vi "Instrument_IO Shift Variables.vi"(8 "error in":errorcluster, 11 "Main Config File Refnum":T1) -> (0 "error out":errorcluster, 3 "VARS Instrument_IO":T2={"error"={"status"=FALSE, "code"=0, "source"=""}, "AI_Tasks_State"=enum."Idle", "AO_Tasks_State"=enum."Idle", "RUN_PMT_AI"=FALSE, "RUN_PMT_AO"=FALSE, "RUN_PMT_DI"=FALSE, "WDT Time Stamp 1"=timestamp(0 s since 1904-01-01), "WDT Time Stamp 2"=timestamp(0 s since 1904-01-01), "RT_TO"=0, "WDT_TO"=0.0, "AO Tasks"=[], "DI Tasks"=[], "Tag Set Directory"=path "c:/ni-rt/startup/tagset", "LogPath"=path "", "DI_Tasks_State"=enum."Idle", "DO Tasks"=[], "RUN_PMT_DO"=FALSE, "DO_Tasks_State"=enum."Idle", "LogErrors?"=FALSE, "System Type"="", "AI Sample Rate"=0.0, "Timed Loop Rate"=0.0, "AI Averaging On"=FALSE, "Agilent Visa Resource"="Agilent", "FEM Visa Resource"="Agilent", "AI Tasks"=""} {"WDT_TO" format="%_4g"})   [LabVIEW 2018]
uses:
  Instrument_IO Shift Variables.ctl
  Common/Module Manager/MM_Module_Action.ctl
  <vilib>/Utility/config.llb/Config Data RefNum.ctl
  Common/COMM_Queues/Command Queue Cluster.ctl
  <vilib>/Utility/config.llb/Read Key (Double).vi
  <vilib>/Utility/config.llb/Read Key (String).vi
  <vilib>/Utility/config.llb/NI_LVConfig.lvlib
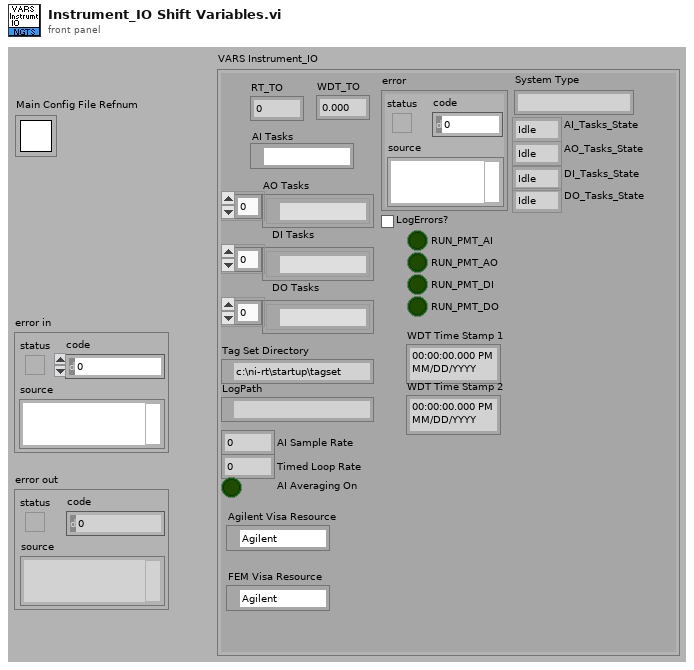
[diagram p1: front panel]
types:
  T1 = typedef "NI_LVConfig.lvlib/Config Data RefNum.ctl" = refnum<k1>
  T2 = typedef "Instrument_IO Shift Variables.ctl" = cluster{"error":errorcluster, "AI_Tasks_State":T3, "AO_Tasks_State":T3, "RUN_PMT_AI":bool, "RUN_PMT_AO":bool, "RUN_PMT_DI":bool, "WDT Time Stamp 1":timestamp, "WDT Time Stamp 2":timestamp, "RT_TO":i32, "WDT_TO":dbl, "AO Tasks":refnum<k21>[], "DI Tasks":refnum<k21>[], "Tag Set Directory":path, "LogPath":path, "DI_Tasks_State":T3, "DO Tasks":refnum<k21>[], "RUN_PMT_DO":bool, "DO_Tasks_State":T3, "LogErrors?":bool, "System Type":string, "AI Sample Rate":dbl, "Timed Loop Rate":dbl, "AI Averaging On":bool, "Agilent Visa Resource":refnum<visa-resource-name>, "FEM Visa Resource":refnum<visa-resource-name>, "AI Tasks":refnum<k21>}
  T3 = typedef "MM_Module_Action.ctl" = enum16{"Idle", "Start", "Run", "Exit"}
  T4 = typedef "Command Queue Cluster.ctl" = cluster{"Command":string, "Variant Data":variant}
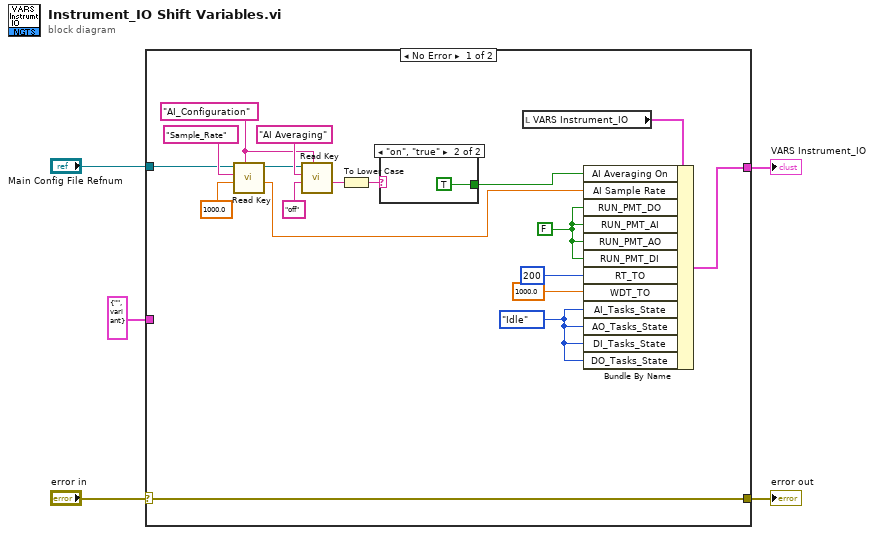
[diagram p0: block diagram]
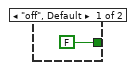
[diagram p2: hidden frame]
diagram:
  n1 = case shown="No Error" "error in" {
    selector: "error in" -> [w22 w26]
    tunnel: [w23 _] -> w5
    tunnel: [w22 w26] -> w3
    tunnel: "Main Config File Refnum" -> [w14 _]
    tunnel: T4 {"Command"="", "Variant Data"=variant} ("queue data") -> [_ _]
    frame No Error {
      w18 = MM_Module_Action."Idle" ("AI_Tasks_State")
      w10 = "AI_Configuration"
      w17 = FALSE
      n2 = call-poly <vilib>:"Read Key.vi"("section"=w10, "default value"=1000.0, "key"="Sample_Rate", "refnum"=w14) -> ("value"=w6:dbl, "refnum out"=w12:T1)  [unwired: 4 in, 2 out]
      n3 = call-poly <vilib>:"Read Key.vi"("section"=w10, "default value"="off", "key"="AI Averaging", "refnum"=w12) -> ("value"=w9:string)  [unwired: 4 in, 3 out]
      n4 = To Lower Case(string=w9) -> (all lower case string=w8:string)
      n5 = case shown="\"on\", \"true\"" w8 {
        tunnel: [FALSE ("AI Averaging On") TRUE ("AI Averaging On")] -> w7
        frame "off", Default {
        }
        frame "on", "true" {
        }
      }
      n6 = local read "VARS Instrument_IO"() -> (w19:T2)
      n7 = Bundle By Name(cluster=w19, "AI Averaging On"=w7, "AI Sample Rate"=w6, "RUN_PMT_DO"=w17, "RUN_PMT_AI"=w17, "RUN_PMT_AO"=w17, "RUN_PMT_DI"=w17, "RT_TO"=200 ("Q_TO"), "WDT_TO"=1000.0, "AI_Tasks_State"=w18, "AO_Tasks_State"=w18, "DI_Tasks_State"=w18, "DO_Tasks_State"=w18) -> (w23:T2)
    }
    frame Error {
    }
  }
  "VARS Instrument_IO" <- w5
  "error out" <- w3
